vi "1259_usbCommand.vi"(8 "error in (no error)":errorcluster, 10 "write buffer":string, 11 "VISA resource name in":refnum<visa-resource-name>) -> (0 "error out":errorcluster, 3 "VISA resource name out":refnum<visa-resource-name>)   [LabVIEW 2018]
uses:
  <vilib>/Instr/_visa.llb/VISA Configure Serial Port (Instr).vi
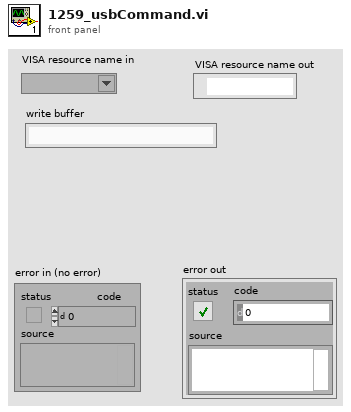
[diagram p1: front panel]
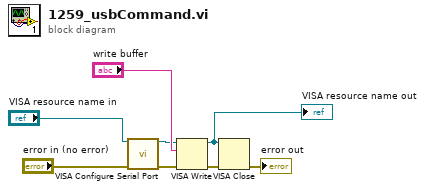
[diagram p0: block diagram]
diagram:
  n1 = call-poly "VISA Configure Serial Port"("VISA resource name"="VISA resource name in", "error in (no error)"="error in (no error)") -> ("VISA resource name out"=w4:refnum<visa-resource-name>, "error out"=w3:errorcluster)  [unwired: 12 in]
  n2 = VISA Write(VISA resource name=w4, write buffer="write buffer", error in (no error)=w3) -> (VISA resource name out=w1:refnum<visa-resource-name>, error out=w5:errorcluster)  [unwired: 1 out]
  "VISA resource name out" <- w1
  n3 = VISA Close(VISA resource name=w1, error in (no error)=w5) -> (error out=→"error out":errorcluster)
